vi "vyezd.vi"   [LabVIEW 2017]
uses:
  <vilib>/myRIO/Instrument Drivers/Onboard IO/PWM/typedefs/PWM Reference.ctl
  <vilib>/myRIO/Common/Instrument Driver Framework/Utilities/typedefs/myRIO Generic Hardware Reference.ctl
  <vilib>/myRIO/Common/Instrument Driver Framework/Utilities/typedefs/Hardware Version Enum.ctl
  <vilib>/myRIO/Common/Instrument Driver Framework/Utilities/typedefs/myRIO v1.0 Reference.ctl
  <vilib>/myRIO/Common/Instrument Driver Framework/Utilities/typedefs/Generic FPGA Reference.ctl
  <vilib>/myRIO/Common/Instrument Driver Framework/myRIO v1.0/PWM/typedefs/PWM Channels Enum.ctl
  <vilib>/myRIO/Instrument Drivers/Onboard IO/PWM/typedefs/PWM Configuration.ctl
  <vilib>/userdefined/High Color/nirio_resource_hc.ctl
  <vilib>/myRIO/Instrument Drivers/Onboard IO/DIO/typedefs/DIO Reference.ctl
  <vilib>/myRIO/Common/Instrument Driver Framework/myRIO v1.0/DIO/typedefs/DIO Channels List.ctl
  <vilib>/myRIO/Common/Instrument Driver Framework/myRIO v1.0/DIO/typedefs/DIO Channels Enum.ctl
  <vilib>/myRIO/Common/Instrument Driver Framework/Utilities/vis/Is FPGA Ref Available.vi
  <vilib>/myRIO/Common/Instrument Driver Framework/myRIO v1.0/PWM/vis/myRIO v1.1 Open PWM.vi
  <vilib>/myRIO/Instrument Drivers/Onboard IO/PWM/vis/Set Duty Cycle and Frequency.vi
  <vilib>/myRIO/Common/Instrument Driver Framework/myRIO v1.0/DIO/vis/myRIO v1.1 Open DIO.vi
  <vilib>/myRIO/Instrument Drivers/Onboard IO/DIO/vis/Write.vi
  <vilib>/myRIO/Common/Instrument Driver Framework/Utilities/vis/Validate Channels.vi
  <vilib>/myRIO/Common/Instrument Driver Framework/myRIO v1.0/PWM/vis/myRIO v1.0 Reserve PWM.vi
  <vilib>/myRIO/Common/Instrument Driver Framework/myRIO v1.0/DIO/vis/myRIO v1.0 Reserve DIO.vi
  <vilib>/myRIO/Common/Instrument Driver Framework/myRIO v1.0/PWM/vis/myRIO v1.0 Build MUX Configuration PWM.vi
  <vilib>/myRIO/Common/Instrument Driver Framework/myRIO v1.0/Resource Manager/vis/myRIO v1.0 Reserve Channel List.vi
  <vilib>/myRIO/Common/Instrument Driver Framework/myRIO v1.0/DIO/vis/myRIO v1.0 Build MUX Configuration DIO.vi
  <vilib>/myRIO/Common/Instrument Driver Framework/myRIO v1.0/Resource Manager/vis/myRIO v1.0 Create Configuration List.vi
  <vilib>/myRIO/Common/Instrument Driver Framework/myRIO v1.0/Resource Manager/vis/myRIO v1.0 Reserve Channel.vi
  <vilib>/myRIO/Common/Instrument Driver Framework/myRIO v1.0/Resource Manager/vis/myRIO v1.0 Unreserve Channel.vi
  <vilib>/myRIO/Common/Instrument Driver Framework/myRIO v1.0/Resource Manager/vis/myRIO v1.0 Build Mutex Name.vi
  <vilib>/Utility/VariantDataType/GetNumericInfo.vi
  <vilib>/Utility/error.llb/Error Cluster From Error Code.vi
  <vilib>/myRIO/Common/Instrument Driver Framework/myRIO v1.0/myRIO v1.1 Open.vi
  <vilib>/myRIO/Common/Instrument Driver Framework/Utilities/vis/IO Manager.vi
  <vilib>/myRIO/Common/Instrument Driver Framework/Utilities/vis/Configuration Manager.vi
  <vilib>/myRIO/Common/Instrument Driver Framework/myRIO v1.0/Resource Manager/vis/myRIO v1.0 Configure IO.vi
  <vilib>/myRIO/Common/Instrument Driver Framework/myRIO v1.0/myRIO v1.0 Close.vi
  <vilib>/myRIO/Common/Instrument Driver Framework/myRIO v1.0/PWM/vis/myRIO v1.0 Write PWM.vi
  <vilib>/myRIO/Common/Instrument Driver Framework/myRIO v1.0/DIO/vis/myRIO v1.0 Write DIO.vi
  <vilib>/myRIO/Express VI/Onboard IO/PWM/PWM Express VI.xnode
  <vilib>/myRIO/Instrument Drivers/Onboard IO/PWM/vis/myRIO PWM Open.xnode
  <vilib>/myRIO/Express VI/Onboard Devices/LED/LED Express VI.xnode
  <vilib>/myRIO/Instrument Drivers/Onboard IO/DIO/vis/myRIO DIO Open.xnode
  <vilib>/myRIO/Instrument Drivers/Onboard IO/PWM/PWM.lvlib
  <vilib>/myRIO/Instrument Drivers/Onboard IO/DIO/DIO.lvlib
types:
  T1 = typedef "PWM.lvlib/PWM Reference.ctl" = cluster{"myRIO Reference":T2, "PWM Channels Enum":T6, "PWM Configuration":T7}
  T2 = typedef "myRIO Generic Hardware Reference.ctl" = cluster{"myRIO Model":T3, "myRIO Hardware Reference":T4}
  T3 = typedef "Hardware Version Enum.ctl" = enum16{"Unknown", "myRIO-1900", "myRIO-1950", "roboRIO", "NI ELVIS RIO CM"}
  T4 = typedef "myRIO v1.0 Reference.ctl" = cluster{"Generic FPGA Reference":T5, "Allow multiple opens":bool}
  T5 = typedef "Generic FPGA Reference.ctl" = refnum<k20>
  T6 = typedef "PWM Channels Enum.ctl" = enum16{"Not Connected", "C/PWM0", "C/PWM1", "A/PWM0", "A/PWM1", "A/PWM2", "B/PWM0", "B/PWM1", "B/PWM2", "PWM/PWM0", "PWM/PWM1", "PWM/PWM2", "PWM/PWM3", "PWM/PWM4", "PWM/PWM5", "PWM/PWM6", "PWM/PWM7", "PWM/PWM8", "PWM/PWM9"}
  T7 = typedef "PWM.lvlib/PWM Configuration.ctl" = cluster{"Frequency":dbl, "Duty Cycle":dbl}
  T8 = typedef "nirio_resource_hc.ctl" = tag
  T9 = typedef "DIO.lvlib/DIO Reference.ctl" = cluster{"myRIO Reference":T2, "DIO Channels List":T10}
  T10 = typedef "DIO Channels List.ctl" = T11[]
  T11 = typedef "DIO Channels Enum.ctl" = enum16{"Not Connected", "C/DIO0", "C/DIO1", "C/DIO2", "C/DIO3", "C/DIO4", "C/DIO5", "C/DIO6", "C/DIO7", "A/DIO0", "A/DIO1", "A/DIO2", "A/DIO3", "A/DIO4", "A/DIO5", "A/DIO6", "A/DIO7", "A/DIO8", "A/DIO9", "A/DIO10", "A/DIO11", "A/DIO12", "A/DIO13", "A/DIO14", "A/DIO15", "B/DIO0", "B/DIO1", "B/DIO2", "B/DIO3", "B/DIO4", "B/DIO5", "B/DIO6", "B/DIO7", "B/DIO8", "B/DIO9", "B/DIO10", "B/DIO11", "B/DIO12", "B/DIO13", "B/DIO14", "B/DIO15", "LED0", "LED1", "LED2", "LED3", "Button0", "DIO/DIO0", "DIO/DIO1", "DIO/DIO2", "DIO/DIO3", "DIO/DIO4", "DIO/DIO5", "DIO/DIO6", "DIO/DIO7", "DIO/DIO8", "DIO/DIO9", "SPI/CS0", "SPI/CS1", "SPI/CS2", "SPI/CS3", "LED RADIO (Green)", "LED RADIO (Red)", "LED COMM (Green)", "LED COMM (Red)", "LED MODE (Green)", "LED MODE (Red)"}
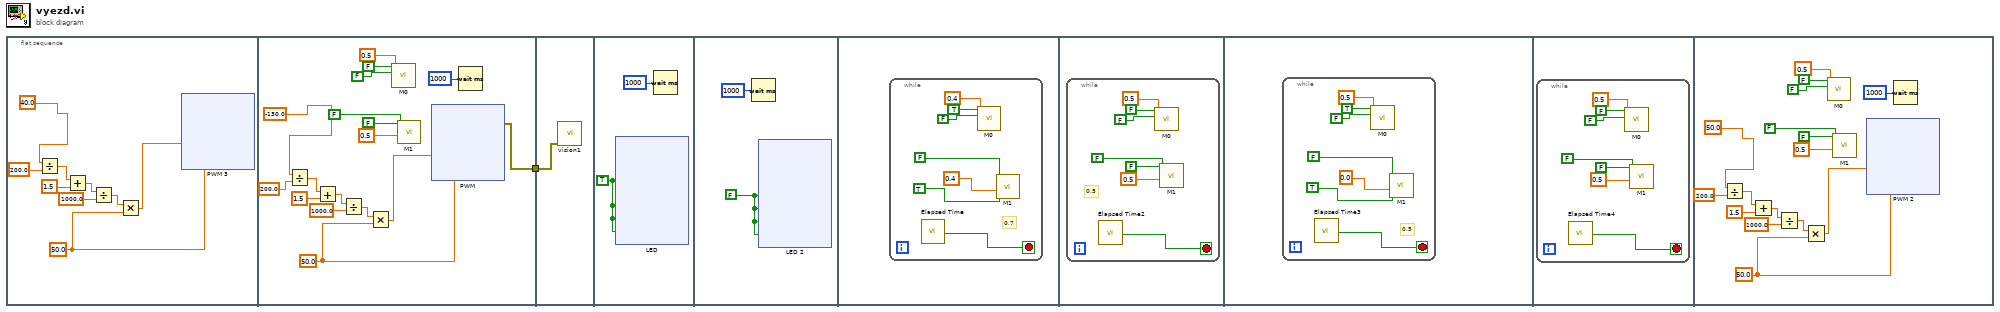
[diagram p0: block diagram]
diagram:
  n1 = flat-sequence {
    tunnel: [w53] -> w1
    tunnel: w1 -> [w98]
    frame #0 {
      w6 = 50.0 ("Frequency [Hz]")
      n2 = Divide(x=40.0, y=200.0) -> (x/y=w9:dbl)
      n3 = Add(x=w9, y=1.5) -> (x+y=w8:dbl)
      n4 = Divide(x=w8, y=1000.0) -> (x/y=w7:dbl)
      n5 = Multiply(x=w7, y=w6) -> (x*y=w10:dbl)
      n6 = xnode "PWM 3"("Duty Cycle"=w10, "Frequency [Hz]"=w6) -> ()  [unwired: 1 in, 1 out]
    }
    frame #1 {
      w58 = 50.0 ("Frequency [Hz]")
      n7 = Divide(x=-130.0, y=200.0) -> (x/y=w61:dbl)
      n8 = Add(x=w61, y=1.5) -> (x+y=w60:dbl)
      n9 = Divide(x=w60, y=1000.0) -> (x/y=w59:dbl)
      n10 = Multiply(x=w59, y=w58) -> (x*y=w62:dbl)
      n11 = call "M0.vi"("Duty Cycle"=0.5, "назад"=FALSE ("вперед"), "вперед"=FALSE ("назад")) -> ()  [unwired: 8 in, 1 out]
      n12 = call "M1.vi"("Duty Cycle"=0.5, "назад"=FALSE ("вперед"), "вперед"=FALSE ("назад")) -> ()  [unwired: 8 in, 1 out]
      n13 = xnode "PWM"("Duty Cycle"=w62, "Frequency [Hz]"=w58) -> ("error out"=w53:errorcluster)  [unwired: 1 in]
      n14 = Wait (ms)(milliseconds to wait=u32 1000) -> ()  [unwired: 1 out]
    }
    frame #2 {
      n15 = call "vision1.vi"("error in"=w98) -> ()  [unwired: 10 in, 1 out]
    }
    frame #3 {
      w100 = TRUE ("LED0")
      n16 = xnode "LED"("LED0"=w100, "LED1"=w100, "LED2"=w100, "LED3"=w100) -> ()  [unwired: 1 in, 1 out]
      n17 = Wait (ms)(milliseconds to wait=u32 1000) -> ()  [unwired: 1 out]
    }
    frame #4 {
      w140 = FALSE ("LED0")
      n18 = Wait (ms)(milliseconds to wait=u32 1000) -> ()  [unwired: 1 out]
      n19 = xnode "LED 2"("LED0"=w140, "LED1"=w140, "LED2"=w140, "LED3"=w140) -> ()  [unwired: 1 in, 1 out]
    }
    frame #5 {
      n20 = while {
        stop <- w185 stop-if-true
        # "0,7"
        n21 = call "Elapsed Time"() -> ("Time has Elapsed"=w185:bool)  [unwired: 12 in, 7 out]
        n22 = call "M0.vi"("Duty Cycle"=0.4, "назад"=FALSE ("вперед"), "вперед"=TRUE ("назад")) -> ()  [unwired: 8 in, 1 out]
        n23 = call "M1.vi"("Duty Cycle"=0.4, "назад"=FALSE ("вперед"), "вперед"=TRUE ("назад")) -> ()  [unwired: 8 in, 1 out]
      }
    }
    frame #6 {
      n24 = while {
        stop <- w192 stop-if-true
        # "0,5"
        n25 = call "Elapsed Time2"() -> ("Time has Elapsed"=w192:bool)  [unwired: 12 in, 7 out]
        n26 = call "M0.vi"("Duty Cycle"=0.5, "назад"=FALSE ("вперед"), "вперед"=FALSE ("назад")) -> ()  [unwired: 8 in, 1 out]
        n27 = call "M1.vi"("Duty Cycle"=0.5, "назад"=FALSE ("вперед"), "вперед"=FALSE ("назад")) -> ()  [unwired: 8 in, 1 out]
      }
    }
    frame #7 {
      n28 = while {
        stop <- w199 stop-if-true
        # "0,5"
        n29 = call "Elapsed Time3"() -> ("Time has Elapsed"=w199:bool)  [unwired: 12 in, 7 out]
        n30 = call "M0.vi"("Duty Cycle"=0.5, "назад"=FALSE ("вперед"), "вперед"=TRUE ("назад")) -> ()  [unwired: 8 in, 1 out]
        n31 = call "M1.vi"("Duty Cycle"=0.0, "назад"=FALSE ("вперед"), "вперед"=TRUE ("назад")) -> ()  [unwired: 8 in, 1 out]
      }
    }
    frame #8 {
      n32 = while {
        stop <- w206 stop-if-true
        n33 = call "Elapsed Time4"() -> ("Time has Elapsed"=w206:bool)  [unwired: 12 in, 7 out]
        n34 = call "M0.vi"("Duty Cycle"=0.5, "назад"=FALSE ("вперед"), "вперед"=FALSE ("назад")) -> ()  [unwired: 8 in, 1 out]
        n35 = call "M1.vi"("Duty Cycle"=0.5, "назад"=FALSE ("вперед"), "вперед"=FALSE ("назад")) -> ()  [unwired: 8 in, 1 out]
      }
    }
    frame #9 {
      w218 = 50.0 ("Frequency [Hz]")
      n36 = Divide(x=50.0, y=200.0) -> (x/y=w221:dbl)
      n37 = Add(x=w221, y=1.5) -> (x+y=w220:dbl)
      n38 = Divide(x=w220, y=1000.0) -> (x/y=w219:dbl)
      n39 = Multiply(x=w219, y=w218) -> (x*y=w222:dbl)
      n40 = call "M0.vi"("Duty Cycle"=0.5, "назад"=FALSE ("вперед"), "вперед"=FALSE ("назад")) -> ()  [unwired: 8 in, 1 out]
      n41 = call "M1.vi"("Duty Cycle"=0.5, "назад"=FALSE ("вперед"), "вперед"=FALSE ("назад")) -> ()  [unwired: 8 in, 1 out]
      n42 = xnode "PWM 2"("Duty Cycle"=w222, "Frequency [Hz]"=w218) -> ()  [unwired: 1 in, 1 out]
      n43 = Wait (ms)(milliseconds to wait=u32 1000) -> ()  [unwired: 1 out]
    }
  }
